vi "main.vi"() -> ()   [LabVIEW 2024]
uses:
  Controls/#typedef_program_data_zadanie_9.ctl
  Controls/#typedef_program_states_calc.ctl
panel:
  out "error out":errorcluster
  in  "error in (no error)":errorcluster
  in  "Program Data":T1
  in  "Stop":bool
  in  "Reset button":bool
  in  "7":bool
  in  "8":bool
  in  "9":bool
  in  "4":bool
  in  "5":bool
  in  "6":bool
  in  "1":bool
  in  "2":bool
  in  "3":bool
  in  "0":bool
  out "Pressed Numbers":string
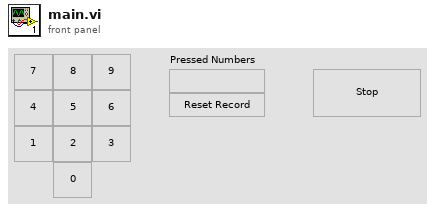
[diagram p1: front panel]
types:
  T1 = typedef "#typedef_program_data_zadanie_9.ctl" = cluster{"Pressed Numbers string":string, "Pressed Numbers char":string}
  T2 = typedef "#typedef_program_states_calc.ctl" = enum16{"Application error", "Init", "Idle", "Button Pressed", "Reset", "Stop"}
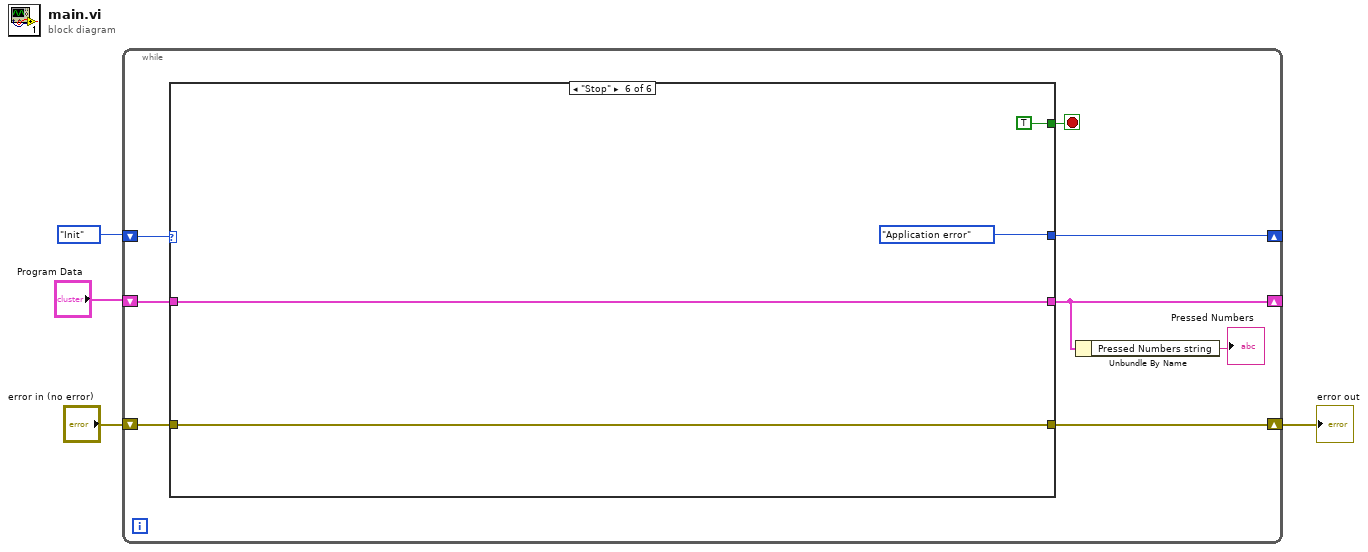
[diagram p0: block diagram]
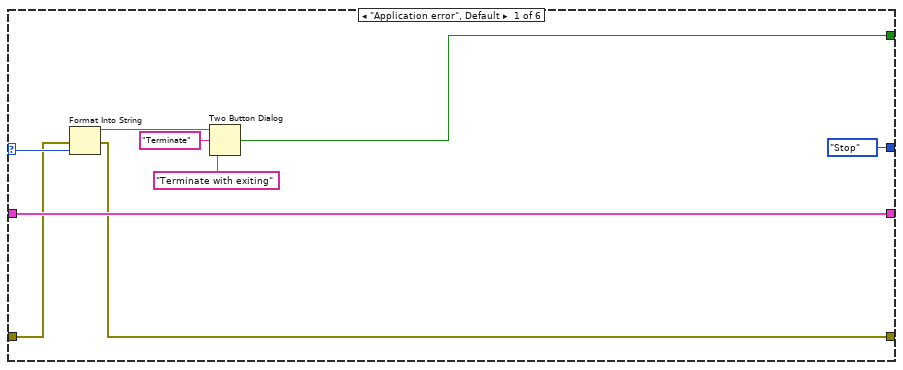
[diagram p2: hidden frame]
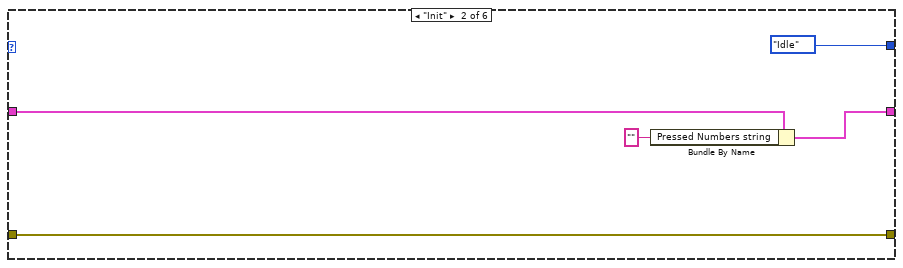
[diagram p3: hidden frame]
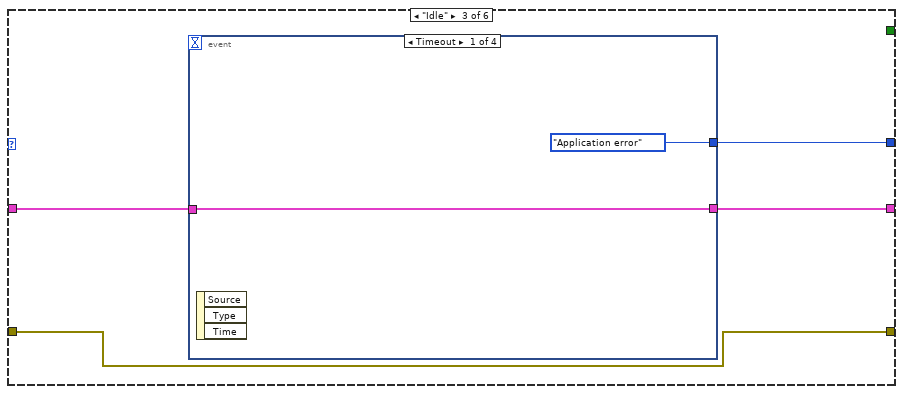
[diagram p4: hidden frame]
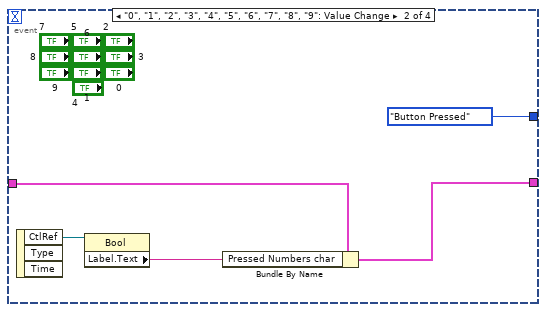
[diagram p5: hidden frame]
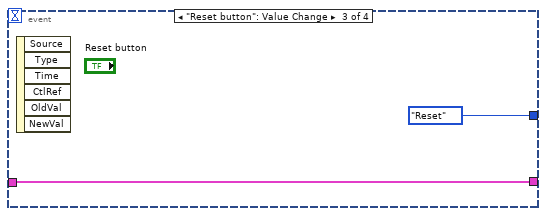
[diagram p6: hidden frame]
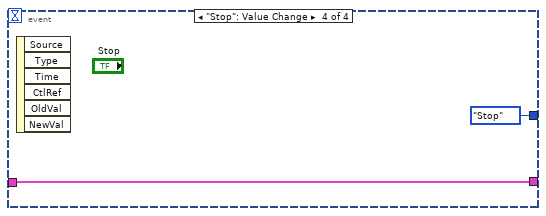
[diagram p7: hidden frame]
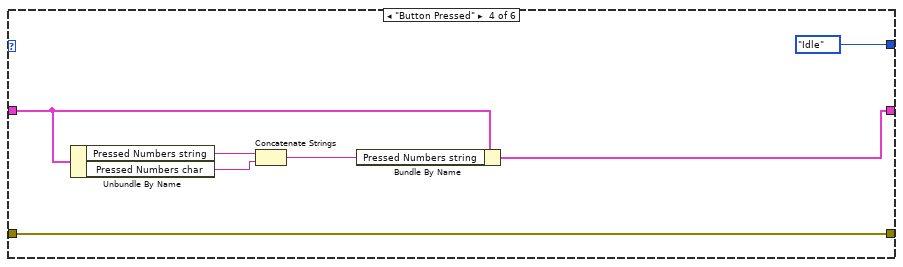
[diagram p8: hidden frame]
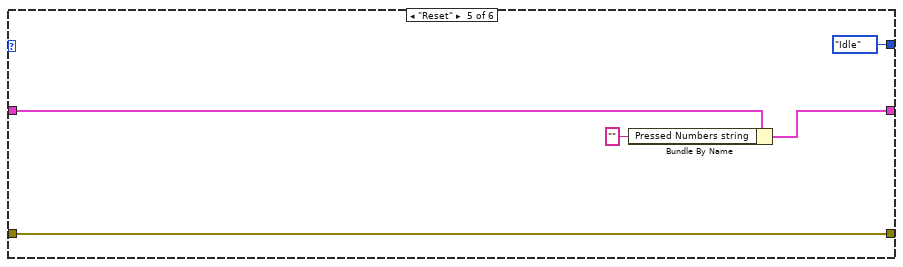
[diagram p9: hidden frame]
diagram:
  n1 = while {
    shift-right: [w11] -> _
    shift-left: #typedef_program_states_calc."Init" ("Enum") -> [w12]
    shift-right: [w8] -> _
    shift-left: "Program Data" -> [w9]
    shift-right: [w5] -> w1
    shift-left: "error in (no error)" -> [w6]
    stop <- w10 stop-if-true
    n2 = case shown="\"Stop\"" w12 {
      selector: w12 -> [w20 _ _ _ _ _]
      tunnel: [#typedef_program_states_calc."Stop" ("Enum") #typedef_program_states_calc."Idle" ("Enum") w30 #typedef_program_states_calc."Idle" ("Enum") #typedef_program_states_calc."Idle" ("Enum") #typedef_program_states_calc."Application error" ("Enum")] -> w11
      tunnel: [w16 _ _ _ _ TRUE] -> w10
      tunnel: w9 -> [w15 w25 w28 w47 w52 w55]
      tunnel: [w15 w23 w29 w43 w51 w55] -> w8
      tunnel: w6 -> [w14 w22 w27 w42 w49 w54]
      tunnel: [w13 w22 w27 w42 w49 w54] -> w5
      frame "Application error", Default {
        n3 = Format Into String(error in=w14, w20) -> (resulting string=w19:string, error out=w13:errorcluster)  [unwired: 2 in]
        n4 = Two Button Dialog(message=w19, 1:"Terminate with exiting" ("F button name (\"Cancel\")"), 2:"Terminate" ("T button name (\"OK\")")) -> (T button?=w16:bool)
      }
      frame "Init" {
        n5 = Bundle By Name(cluster=w25, "Pressed Numbers string"="" ("Pressed Numbers current")) -> (w23:T1)
      }
      frame "Idle" {
        n6 = event shown="[0] Timeout" {
          selector: _ -> [_ _ _ _]
          dyn-events: _ -> [_ _ _ _]
          timeout: _ -> [_ _ _ _]
          tunnel: [#typedef_program_states_calc."Application error" ("Enum") #typedef_program_states_calc."Button Pressed" ("Enum") #typedef_program_states_calc."Reset" ("Enum") #typedef_program_states_calc."Stop" ("Enum")] -> w30
          tunnel: [w31 w35 w38 w40] -> w29
          tunnel: w28 -> [w31 w34 w38 w40]
          event Timeout {
            n7 = event-data() -> ()  [unwired: 1 in, 3 out]
          }
          event "0", "1", "2", "3", "4", "5", "6", "7", "8", "9": Value Change {
            n8 = event-data() -> ("CtlRef"=w37:refnum<vi>)  [unwired: 1 in, 2 out]
            n9 = property class="Bool"(reference=w37) -> ("Label.Text"=w33:string)  [unwired: 1 in, 2 out]
            n10 = Bundle By Name(cluster=w34, "Pressed Numbers char"=w33) -> (w35:T1)
          }
          event "Reset button": Value Change {
            n11 = event-data() -> ()  [unwired: 1 in, 6 out]
          }
          event "Stop": Value Change {
            n12 = event-data() -> ()  [unwired: 1 in, 6 out]
          }
        }
      }
      frame "Button Pressed" {
        n13 = Unbundle By Name(w47) -> ("Pressed Numbers string"=w46:string, "Pressed Numbers char"=w45:string)
        n14 = Concatenate Strings(w46, w45) -> (w44:string)
        n15 = Bundle By Name(cluster=w47, "Pressed Numbers string"=w44) -> (w43:T1)
      }
      frame "Reset" {
        n16 = Bundle By Name(cluster=w52, "Pressed Numbers string"="") -> (w51:T1)
      }
      frame "Stop" {
      }
    }
    n17 = Unbundle By Name(w8) -> ("Pressed Numbers string"=→"Pressed Numbers":string)
  }
  "error out" <- w1
